vi "set keypair mem.vi"(8 "error in":errorcluster, 9 "key":string, 10 "cert":string, 11 "lvlibretls configurable context in":refnum<class "lvlibretls configurable context.lvclass">) -> (0 "error out":errorcluster, 3 "lvlibretls configurable context out":refnum<class "lvlibretls configurable context.lvclass">)   [LabVIEW 2016, in "lvlibretls configurable context.lvclass"]
uses:
  lvlibretls configurable context.lvclass
  lvlibretls configurable context.lvclass/lvlibretls configurable context.ctl
  lv tls dll.lvlib
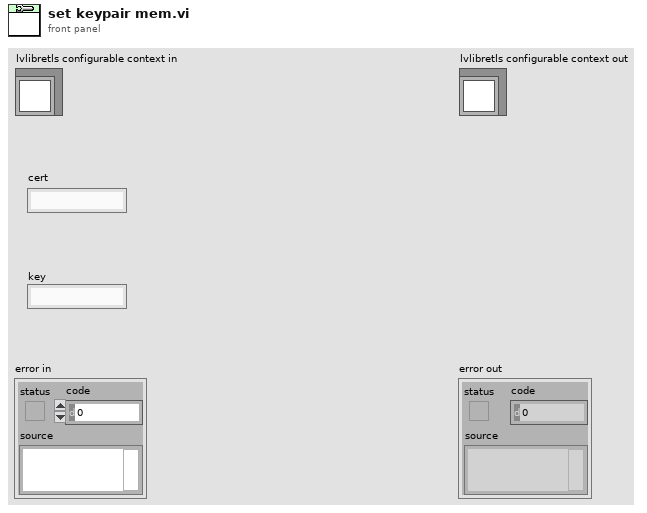
[diagram p1: front panel]
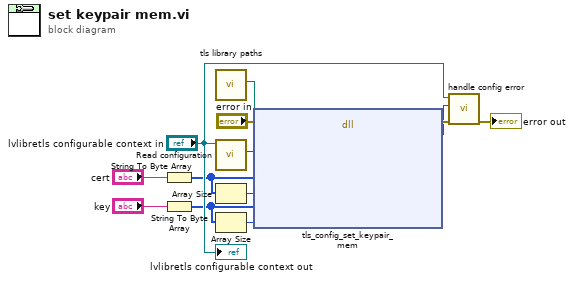
[diagram p0: block diagram]
diagram:
  n1 = String To Byte Array(string="cert") -> (unsigned byte array=w4:u8[])
  n2 = String To Byte Array(string="key") -> (unsigned byte array=w1:u8[])
  n3 = call "tls library paths.vi"() -> ("libtls"=w13:path)  [unwired: 8 in, 3 out]
  n4 = call "Read configuration.vi"("lvlibretls configurable context in"="lvlibretls configurable context in") -> ("configuration"=w12:u64)  [unwired: 10 in]
  n5 = Array Size(array=w4) -> (size(s)=w3:i32)
  n6 = Array Size(array=w1) -> (size(s)=w2:i32)
  n7 = dll-call lib="C:/Users/IEUser/Desktop/tlssimple/libtls-15.dll" fn="tls_config_set_keypair_mem"(path in=w13, error in="error in", "config"=w12, "certfile"=w4, "certlen"=w3, "keyfile"=w1, "keylen"=w2) -> (error out=w11:errorcluster, "return"=w10:i32)  [unwired: 6 in, 1 out]
  n8 = call "handle config error.vi"("error in"=w11, "return"=w10, "lvlibretls configurable context in"="lvlibretls configurable context in") -> ("error out"=→"error out":errorcluster)  [unwired: 8 in]
  "lvlibretls configurable context out" <- "lvlibretls configurable context in"
